vi "Launch Once.vi"(6 "Shutdown if running":bool, 8 "error in (no error)":errorcluster, 11 "Parallel Process in":refnum<class "Parallel Process.lvclass">) -> (0 "error out":errorcluster, 3 "Parallel Process out":refnum<class "Parallel Process.lvclass">)   [LabVIEW 2011, in "Messenging.lvlib" / "Parallel Process.lvclass"]
doc: "Launches the Parallel Process the fisrt call, then returns that same process with each subsequent call.\n\nThis VI is reentrant (preallocated clones) so can hold a different PP at each location in that it is used."
uses:
  Parallel Process.lvclass
panel:
  # "Launches the Parallel Process the fisrt call, then returns that same process with each subsequent call.\n\nThis VI is reentrant (preallocated clones) so can hold a different PP at each location in that it is used."
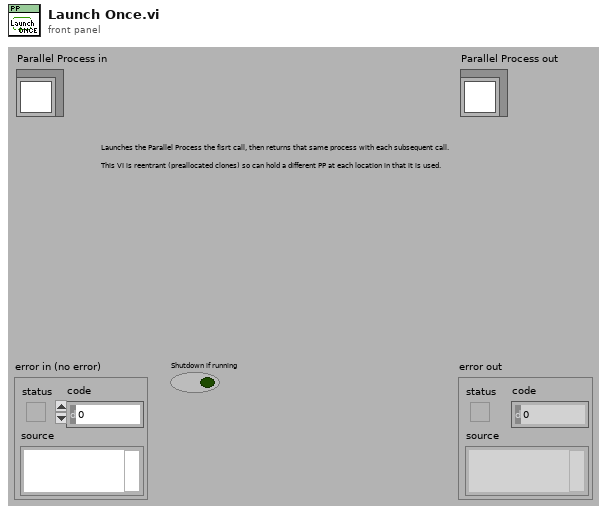
[diagram p1: front panel]
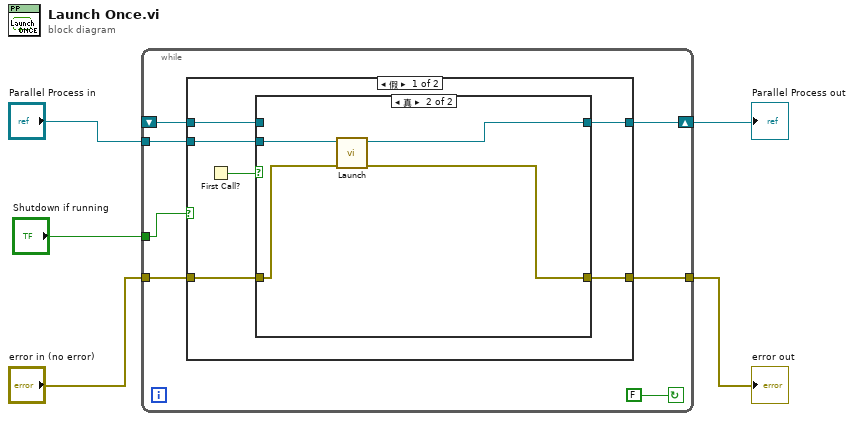
[diagram p0: block diagram]
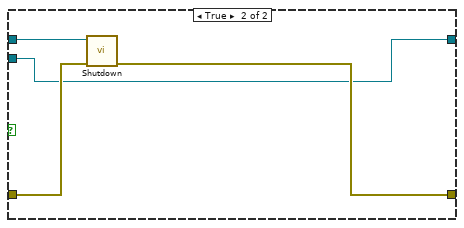
[diagram p3: hidden frame]
diagram:
  n1 = while {
    shift-right: [w11] -> w4
    shift-left: _ -> [w10]
    tunnel: "Parallel Process in" -> [w12]
    tunnel: "Shutdown if running" -> [w8]
    tunnel: "error in (no error)" -> [w7]
    tunnel: [w6] -> w1
    stop <- FALSE continue-if-true
    n2 = case shown="假" w8 {
      tunnel: w12 -> [w18 w25]
      tunnel: [w17 w25] -> w11
      tunnel: w10 -> [w16 w26]
      tunnel: w7 -> [w14 w28]
      tunnel: [w13 w27] -> w6
      frame False {
        n3 = First Call?() -> (First Call?: T/F=w15:bool)
        n4 = case shown="真" w15 {
          tunnel: w18 -> [_ w24]
          tunnel: [w20 w23] -> w17
          tunnel: w16 -> [w20 _]
          tunnel: w14 -> [w19 w22]
          tunnel: [w19 w21] -> w13
          frame False {
          }
          frame True {
            n5 = call-dynamic "Launch.vi"("error in"=w22, "Parallel Process in"=w24) -> ("error out"=w21:errorcluster, "Parallel Process out"=w23:refnum<class "Parallel Process.lvclass">)  [unwired: 3 in, 5 out]
          }
        }
      }
      frame True {
        n6 = call-dynamic "Shutdown.vi"("error in (no error)"=w28, "Parallel Process in"=w26) -> ("error out"=w27:errorcluster)  [unwired: 2 in, 7 out]
      }
    }
  }
  "error out" <- w1
  "Parallel Process out" <- w4
